vi "Measure.vi"(0 "VISA resource name":refnum<visa-resource-name>, 5 "Function Mode String":string, 7 "Function Mode Numeric":u8(ring) items=["MANU", "AUTO"], 9 "Step number for Auto Mode":u8(ring)=1 items=["16"=16, "15"=15, "14"=14, "13"=13, "12"=12, "11"=11, "10"=10, "9"=9, "8"=8, "7"=7, "6"=6, "5"=5, "4"=4, "3"=3, "2"=2, "1"=1], 11 "error in":errorcluster) -> (4 "VISA resource name out":refnum<visa-resource-name>, 6 "Return  the test status":string, 10 "Return the String Count":u16, 15 "error out":errorcluster)   [LabVIEW 2021, in "GPT-9000.lvlib"]
uses:
  GPT-9000.lvlib
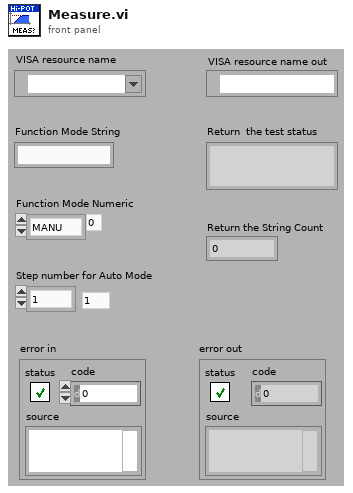
[diagram p1: front panel]
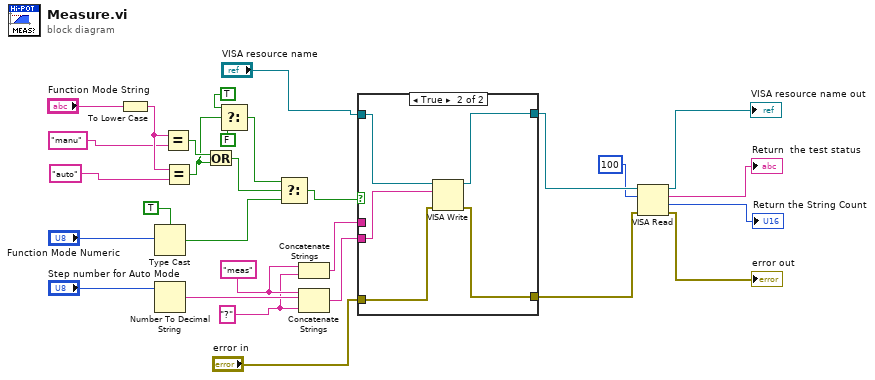
[diagram p0: block diagram]
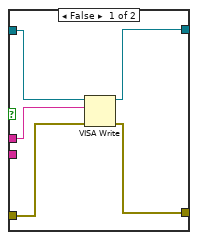
[diagram p2: hidden frame]
diagram:
  w14 = "?" ("string")
  w15 = "meas" ("string")
  n1 = To Lower Case(string="Function Mode String") -> (all lower case string=w28:string)
  n2 = Type Cast(type=TRUE, x="Function Mode Numeric") -> (*(type *) &x=w18:bool)
  n3 = Number To Decimal String(number="Step number for Auto Mode") -> (decimal integer string=w16:string)  [unwired: 1 in]
  n4 = Equal?(x=w28, y="manu") -> (x = y?=w22:bool)
  n5 = Equal?(x=w28, y="auto") -> (x = y?=w1:bool)
  n6 = Or(x=w22, y=w1) -> (x .or. y?=w23:bool)
  n7 = Select(t=TRUE, s=w1, f=FALSE) -> (s? t:f=w19:bool)
  n8 = Select(t=w19, s=w23, f=w18) -> (s? t:f=w13:bool)
  n9 = Concatenate Strings(w15, w14) -> (w10:string)
  n10 = Concatenate Strings(w15, w16, w14) -> (w9:string)
  n11 = case shown="True" w13 {
    tunnel: "VISA resource name" -> [w34 w39]
    tunnel: "error in" -> [w31 w38]
    tunnel: w10 -> [w30 _]
    tunnel: w9 -> [_ w35]
    tunnel: [w33 w37] -> w8
    tunnel: [w32 w36] -> w7
    frame False {
      n12 = VISA Write(VISA resource name=w34, write buffer=w30, error in (no error)=w31) -> (VISA resource name out=w33:refnum<visa-resource-name>, error out=w32:errorcluster)  [unwired: 1 out]
    }
    frame True {
      n13 = VISA Write(VISA resource name=w39, write buffer=w35, error in (no error)=w38) -> (VISA resource name out=w37:refnum<visa-resource-name>, error out=w36:errorcluster)  [unwired: 1 out]
    }
  }
  n14 = VISA Read(VISA resource name=w8, byte count=u32 100, error in (no error)=w7) -> (VISA resource name out=→"VISA resource name out":refnum<visa-resource-name>, read buffer=→"Return  the test status":string, return count=→"Return the String Count":u32, error out=→"error out":errorcluster)
